vi "merge all hydrolysis.vi"(6 "merge_preexisting":bool, 7 "current_starttime":i32, 8 "error in (no error)":errorcluster, 9 "simulation_starttime":i32, 10 "reactor_names":string, 11 "working_dir":string) -> (0 "error out":errorcluster)   [LabVIEW 2019, in "libFileFunctions.lvlib"]
doc: "void merge_all_hydrolysis(const char* working_dir, const char* reactor_names, int simulation_starttime, int current_starttime);"
uses:
  libFileFunctions.lvlib
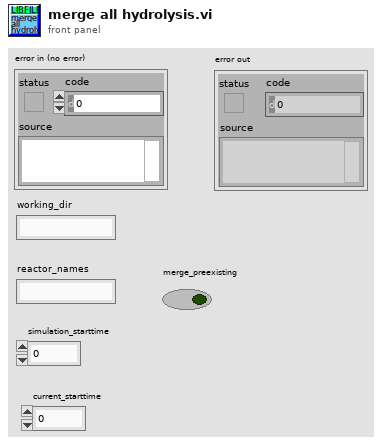
[diagram p1: front panel]
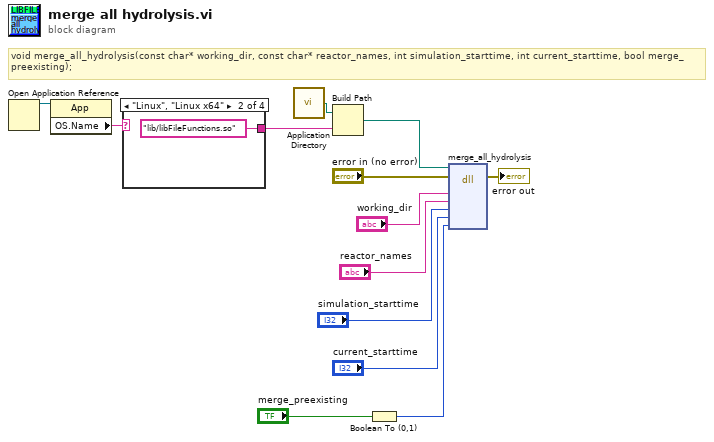
[diagram p0: block diagram]
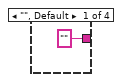
[diagram p2: hidden frame]
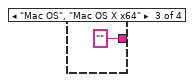
[diagram p3: hidden frame]
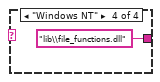
[diagram p4: hidden frame]
diagram:
  # "void merge_all_hydrolysis(const char* working_dir, const char* reactor_names, int simulation_starttime, int current_starttime, bool merge_preexisting);"
  n1 = Open Application Reference() -> (3:w7:refnum<vi>)  [unwired: 4 in, 1 out]
  n2 = property class="App"(reference=w7) -> ("OS.Name"=w6:string)  [unwired: 1 in, 2 out]
  n3 = case shown="\"Linux\", \"Linux x64\"" w6 {
    tunnel: ["" ("return type") "lib/libFileFunctions.so" ("name or relative path") "" ("return type") "lib\\file_functions.dll" ("name or relative path")] -> w5
    frame "", Default {
    }
    frame "Linux", "Linux x64" {
    }
    frame "Mac OS", "Mac OS X x64" {
    }
    frame "Windows NT" {
    }
  }
  n4 = call <vilib>:"Application Directory.vi"() -> ("Application Directory"=w4:path)
  n5 = Build Path(base path=w4, name or relative path=w5) -> (appended path=w3:path)
  n6 = Boolean To (0,1)(Boolean="merge_preexisting") -> (0, 1=w1:i16)
  n7 = dll-call lib="home/paul/Schreibtisch/Biogas_plant_setup/LabView/lib/libFileFunctions/libFileFunctions.*" fn="merge_all_hydrolysis"(path in=w3, error in="error in (no error)", "working_dir"="working_dir", "reactor_names"="reactor_names", "simulation_starttime"="simulation_starttime", "current_starttime"="current_starttime", "merge_preexisting"=w1) -> (error out=→"error out":errorcluster)  [unwired: 7 in, 1 out]
